vi "Reset.vi"(8 "error in (no error)":errorcluster, 11 "VISA resource name":refnum<visa-resource-name>) -> (0 "error out":errorcluster, 3 "VISA resource name out":refnum<visa-resource-name>)   [LabVIEW 2010, in "Temptronic TP04300.lvlib"]
doc: "This VI resets the instrument to the Cycle screen. Any device-specific errors, the uppper and lower temperature limits are reset. System switches to the air mode and sets the test time to 0(zero) seconds. If the system was cycling or controlling at temperature, the air flow shuts off and cycling is interrupted. Setpoint number 5 becomes the selected setpoint. \n\nNote: After sending this command, wait 4 seconds before sending another command"
uses:
  Temptronic TP04300.lvlib
  Instance           1 13Saved   Reset .vi
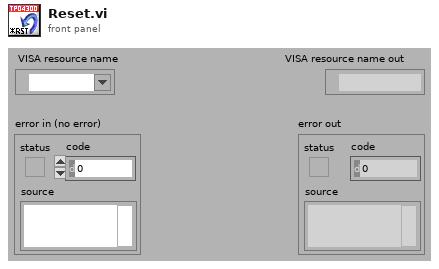
[diagram p1: front panel]
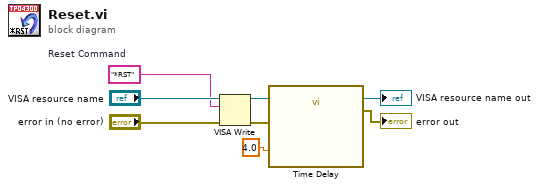
[diagram p0: block diagram]
diagram:
  w5 = "*RST"  # Reset Command
  n1 = VISA Write(VISA resource name="VISA resource name", write buffer=w5, error in (no error)="error in (no error)") -> (VISA resource name out=→"VISA resource name out":refnum<visa-resource-name>, error out=w3:errorcluster)  [unwired: 1 out]
  n2 = call "Time Delay"("error in (no error)"=w3, "Delay Time (s)"=4.0) -> ("error out"=→"error out":errorcluster)  [unwired: 9 in]
